vi "Write 1D Array DBL.vi"(8 "error in (no error)":errorcluster, 9 "start index (0)":i64, 10 "value":dbl[](array[numeric]), 11 "pointer in":u64) -> (0 "error out":errorcluster, 1 "start index out":i64, 2 "number of elements":i64, 3 "pointer out":u64)   [LabVIEW 2013, in "Linux RT IPC.Shared Memory.lvlib"]
uses:
  Linux RT IPC.Shared Memory.lvlib
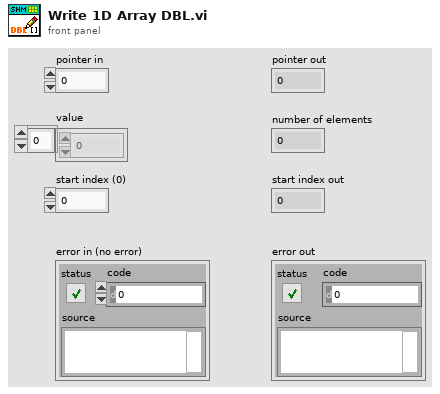
[diagram p1: front panel]
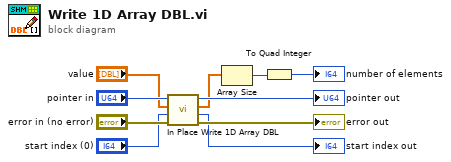
[diagram p0: block diagram]
diagram:
  n1 = call "In Place Write 1D Array DBL.vi"("error in (no error)"="error in (no error)", "start index (0)"="start index (0)", "values in"="value", "pointer in"="pointer in") -> ("error out"=→"error out":errorcluster, "start index out"=→"start index out":i64, "values out"=w1:dbl[], "pointer out"=→"pointer out":u64)  [unwired: 4 in]
  n2 = Array Size(array=w1) -> (size(s)=w2:i32)
  n3 = To Quad Integer(1:w2) -> (0:→"number of elements":i64)
